vi "Obtain Request Events.vi"(8 "error in (no error)":errorcluster, 10 "Create New? (F)":bool) -> (0 "error out":errorcluster, 2 "Acquisition Request Events":T1)   [LabVIEW 2019, in "Acquisition.lvlib"]
doc: "This VI Obtains/Creates the Requests events that will be used for other modules to communicate with the module that owns this VI. These Requests events will be accessed only via Public API methods for this module.\n\n<b>NOTE</b>: The contents of this VI are automatically generated and modified by the <b>Tools > Delacor > DQMH</b> utilities. Consider using those utilities instead of making your own modifications to this VI.\n_____\nBased on Delacor QMH Project Template 4.0.0.47.\n_____\nBased on DQMH Project Template 6.1.0.94."
uses:
  Acquisition.lvlib
  Request Events--cluster.ctl
  Stop Argument--cluster.ctl
  Show Panel Argument--cluster.ctl
  Hide Panel Argument--cluster.ctl
  Get Module Execution Status Argument--cluster.ctl
  Show Diagram Argument--cluster.ctl
  Stop Acquiring Argument--cluster.ctl
  Wakeup Helper Loop Argument--cluster.ctl
  WiBCI16T_Data.ctl
  WiBCI16T_Status.ctl
  Reg_Map.ctl
  Acquisition Types.ctl
  Change Settings Argument--cluster.ctl
  Signal Type--enum.ctl
  Calibration Values--cluster.ctl
  Calibrate DAQ Argument--cluster.ctl
  Start Acquiring Argument--cluster.ctl
  Start Acquiring (Reply Payload)--cluster.ctl
  Command_TestData Argument--cluster.ctl
  Check WiFi AP Argument--cluster.ctl
  Command_NoiseData Argument--cluster.ctl
  Command_LiveData Argument--cluster.ctl
  Command_ImpedanceData Argument--cluster.ctl
  Command_GoToIdle Argument--cluster.ctl
  Soft Trigger Argument--cluster.ctl
  Start IMP Acquiring Argument--cluster.ctl
  Stop IMP acquiring Argument--cluster.ctl
  Start GND Loop acquiring Argument--cluster.ctl
  IMP data updated Argument--cluster.ctl
  IMP data updated (Reply Payload)--cluster.ctl
  Start CNV Acquiring Argument--cluster.ctl
  Start EOC Acquiring Argument--cluster.ctl
  Wake-up Helper Loop for Pkt Loss Calc Argument--cluster.ctl
  Stop Pkt Loss Calc Argument--cluster.ctl
  Update Packet ID Argument--cluster.ctl
  Calculate Packet Loss Argument--cluster.ctl
  Command_GndImpedanceData Argument--cluster.ctl
panel:
  # "NOTE: The contents of this VI are automatically generated and modified by the Tools > Delacor > DQMH utilities. Consider using those utilities instead of making your own modifications to this VI."
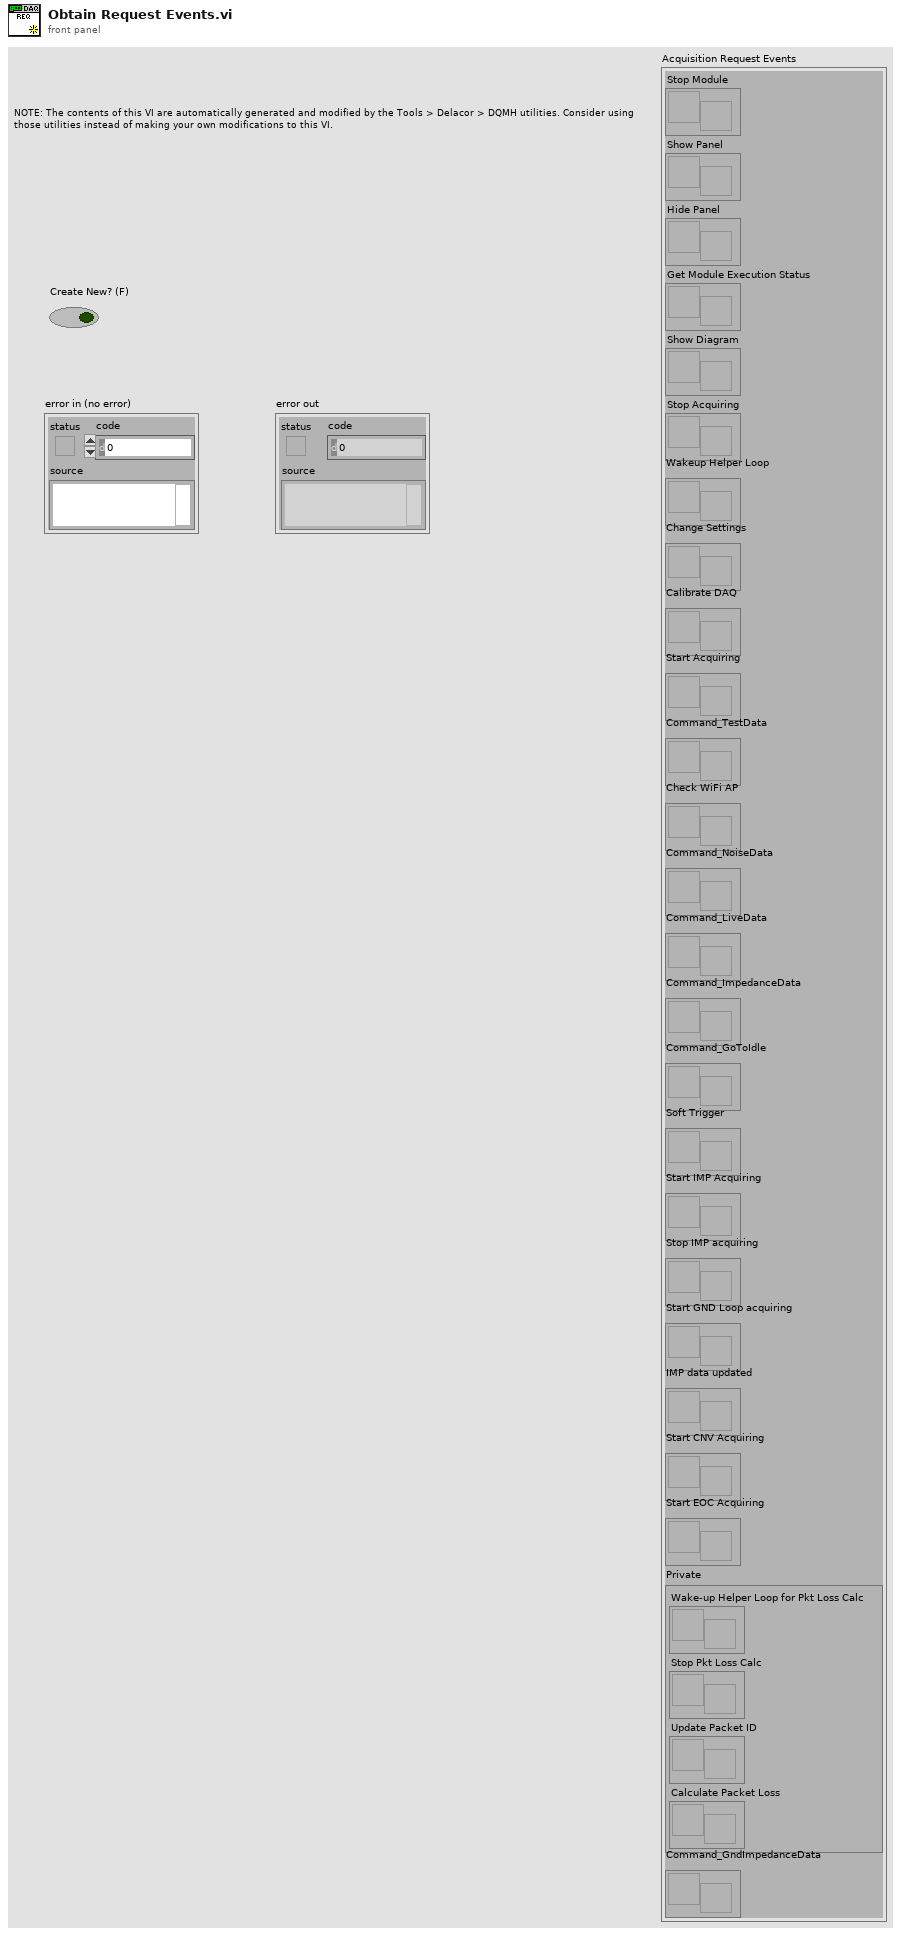
[diagram p1: front panel]
types:
  T1 = typedef "Acquisition.lvlib/Request Events--cluster.ctl" = cluster{"Stop Module":refnum<user-event>, "Show Panel":refnum<user-event>, "Hide Panel":refnum<user-event>, "Get Module Execution Status":refnum<user-event>, "Show Diagram":refnum<user-event>, "Stop Acquiring":refnum<user-event>, "Wakeup Helper Loop":refnum<user-event>, "Change Settings":refnum<user-event>, "Calibrate DAQ":refnum<user-event>, "Start Acquiring":refnum<user-event>, "Command_TestData":refnum<user-event>, "Check WiFi AP":refnum<user-event>, "Command_NoiseData":refnum<user-event>, "Command_LiveData":refnum<user-event>, "Command_ImpedanceData":refnum<user-event>, "Command_GoToIdle":refnum<user-event>, "Soft Trigger":refnum<user-event>, "Start IMP Acquiring":refnum<user-event>, "Stop IMP acquiring":refnum<user-event>, "Start GND Loop acquiring":refnum<user-event>, "IMP data updated":refnum<user-event>, "Start CNV Acquiring":refnum<user-event>, "Start EOC Acquiring":refnum<user-event>, "Private":cluster{"Wake-up Helper Loop for Pkt Loss Calc":refnum<user-event>, "Stop Pkt Loss Calc":refnum<user-event>, "Update Packet ID":refnum<user-event>, "Calculate Packet Loss":refnum<user-event>}, "Command_GndImpedanceData":refnum<user-event>}
  T2 = typedef "Acquisition.lvlib/Command_GndImpedanceData Argument--cluster.ctl" = cluster{"Boolean":bool}
  T3 = typedef "Acquisition.lvlib/Calculate Packet Loss Argument--cluster.ctl" = cluster{"Data Array":u32[]}
  T4 = typedef "Acquisition.lvlib/Update Packet ID Argument--cluster.ctl" = cluster{"Packet ID":u32}
  T5 = typedef "Acquisition.lvlib/Stop Pkt Loss Calc Argument--cluster.ctl" = cluster{"Boolean":bool}
  T6 = typedef "Acquisition.lvlib/Wake-up Helper Loop for Pkt Loss Calc Argument--cluster.ctl" = cluster{"Boolean":bool}
  T7 = typedef "Acquisition.lvlib/Start EOC Acquiring Argument--cluster.ctl" = cluster{"Boolean":bool}
  T8 = typedef "Acquisition.lvlib/Start CNV Acquiring Argument--cluster.ctl" = cluster{"Boolean":bool}
  T9 = typedef "Acquisition.lvlib/IMP data updated Argument--cluster.ctl" = cluster{"Wait Notifier":refnum<notifier>, "wait for reply":bool}
  T10 = typedef "Acquisition.lvlib/Start GND Loop acquiring Argument--cluster.ctl" = cluster{"Boolean":bool}
  T11 = typedef "Acquisition.lvlib/Stop IMP acquiring Argument--cluster.ctl" = cluster{"Boolean":bool}
  T12 = typedef "Acquisition.lvlib/Start IMP Acquiring Argument--cluster.ctl" = cluster{"Boolean":bool}
  T13 = typedef "Acquisition.lvlib/Soft Trigger Argument--cluster.ctl" = cluster{"Value":i8}
  T14 = typedef "Acquisition.lvlib/Command_GoToIdle Argument--cluster.ctl" = cluster{"Boolean":bool}
  T15 = typedef "Acquisition.lvlib/Command_ImpedanceData Argument--cluster.ctl" = cluster{"Boolean":bool}
  T16 = typedef "Acquisition.lvlib/Command_LiveData Argument--cluster.ctl" = cluster{"Boolean":bool}
  T17 = typedef "Acquisition.lvlib/Command_NoiseData Argument--cluster.ctl" = cluster{"Boolean":bool}
  T18 = typedef "Acquisition.lvlib/Check WiFi AP Argument--cluster.ctl" = cluster{"Connected ?":bool}
  T19 = typedef "Acquisition.lvlib/Command_TestData Argument--cluster.ctl" = cluster{"Boolean":bool}
  T20 = typedef "Acquisition.lvlib/Start Acquiring Argument--cluster.ctl" = cluster{"Wait Notifier":refnum<notifier>, "wait for reply":bool}
  T21 = typedef "Acquisition.lvlib/Calibrate DAQ Argument--cluster.ctl" = cluster{"None":bool}
  T22 = typedef "Acquisition.lvlib/Change Settings Argument--cluster.ctl" = cluster{"Signal Type":T23, "Calibration Array":T24[]}
  T23 = typedef "Acquisition.lvlib/Signal Type--enum.ctl" = enum16{"Sine Wave", "Square with Noise"}
  T24 = typedef "Acquisition.lvlib/Calibration Values--cluster.ctl" = cluster{"Slope":dbl, "Offset":dbl}
  T25 = typedef "Acquisition.lvlib/Wakeup Helper Loop Argument--cluster.ctl" = cluster{"connection UDP":refnum<k16>, "En MAP":u16, "WiBCI16T Data out":T26, "Acquisition Types":T29}
  T26 = typedef "Acquisition.lvlib/WiBCI16T_Data.ctl" = cluster{"EEG Ch 1":dbl, "EEG Ch 2":dbl, "EEG Ch 3":dbl, "EEG Ch 4":dbl, "EEG Ch 5":dbl, "EEG Ch 6":dbl, "EEG Ch 7":dbl, "EEG Ch 8":dbl, "EEG Ch 9":dbl, "EEG Ch 10":dbl, "EEG Ch 11":dbl, "EEG Ch 12":dbl, "EEG Ch 13":dbl, "EEG Ch 14":dbl, "EEG Ch 15":dbl, "EEG Ch 16":dbl, "X-Accel":i16, "Y-Accel":i16, "Z-Accel":i16, "X-Gyro":i16, "Y-Gyro":i16, "Z-Gyro":i16, "Timer":u32, "Packet ID":u32, "HW Trig1":u8, "SW Trig1":i8, "HW Trig2":u8, "SW Trig2":i8, "WiBCI Status":T27, "Reg Map":T28}
  T27 = typedef "Acquisition.lvlib/WiBCI16T_Status.ctl" = cluster{"Mode Byte":u8, "Ch Config":u8, "Ch Ref Map":u16, "Ch Enable Map":u16, "Temperature":sgl, "Battery":u8, "Version":string}
  T28 = typedef "Acquisition.lvlib/Reg_Map.ctl" = cluster{"ADS1":u8[], "ADS2":u8[]}
  T29 = typedef "Acquisition.lvlib/Acquisition Types.ctl" = cluster{"Acq Types":enum16{"Single Graph", "Eyes O/C", "CNV Demo", "Impedance", "Graph"}}
  T30 = typedef "Acquisition.lvlib/Stop Acquiring Argument--cluster.ctl" = cluster{"Boolean":bool}
  T31 = typedef "Acquisition.lvlib/Hide Panel Argument--cluster.ctl" = cluster{"Hide Panel?":bool}
  T32 = typedef "Acquisition.lvlib/Show Panel Argument--cluster.ctl" = cluster{"Show Panel?":bool}
  T33 = typedef "Acquisition.lvlib/Show Diagram Argument--cluster.ctl" = cluster{"Debug?":bool}
  T34 = typedef "Acquisition.lvlib/Get Module Execution Status Argument--cluster.ctl" = cluster{"Running?":bool}
  T35 = typedef "Acquisition.lvlib/Stop Argument--cluster.ctl" = cluster{"Origin":string, "Exit via Stop Module Req?":bool, "Wait for Module to stop?":bool}
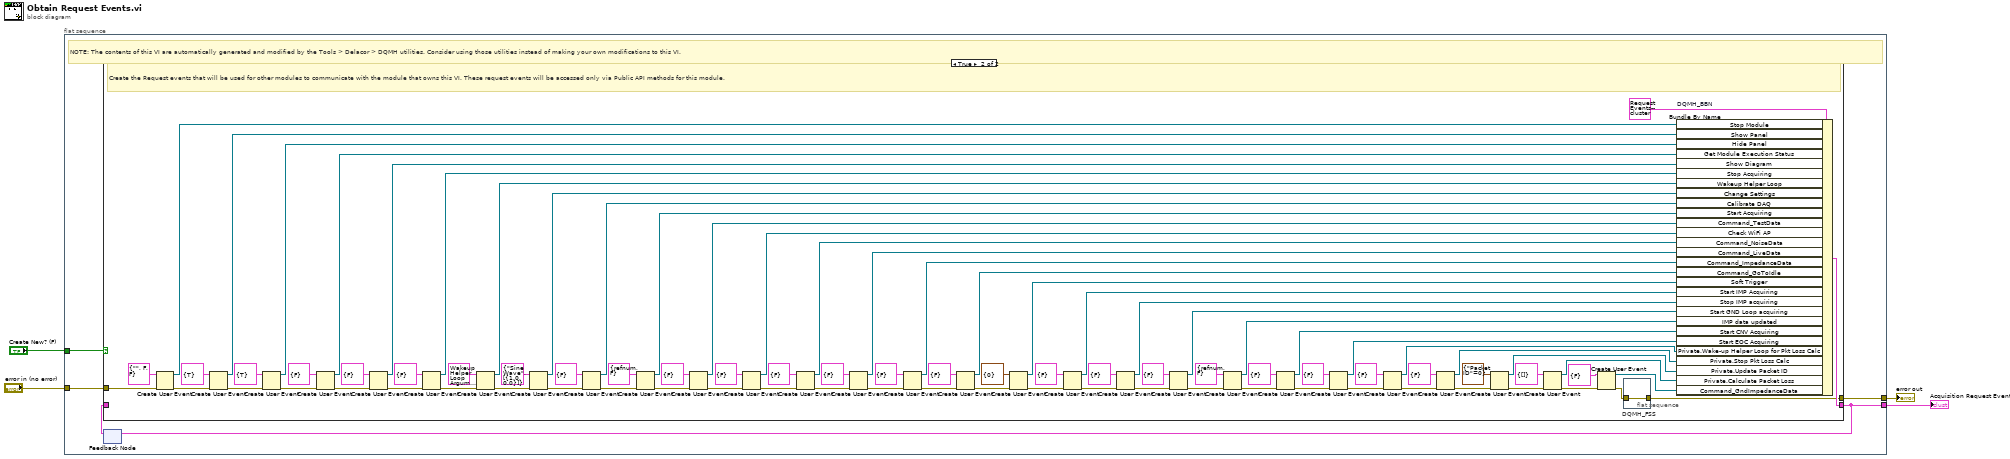
[diagram p0: block diagram]
diagram:
  n1 = flat-sequence {
    tunnel: [w9] -> w4
    tunnel: "error in (no error)" -> [w8]
    tunnel: [w6] -> w2
    tunnel: "Create New? (F)" -> [w5]
    frame #0 {
      # "NOTE: The contents of this VI are automatically generated and modified by the Tools > Delacor > DQMH utilities. Consider using those utilities instead of making your own modifications to this VI."
      n2 = feedback #1() -> (w7:T1)  [unwired: 1 in]
      n3 = case shown="True" w5 {
        tunnel: [w10 w89] -> w9
        tunnel: w8 -> [w10 w99]
        tunnel: [w11 w96] -> w6
        tunnel: w7 -> [w11 _]
        frame False {
          # "Obtain the Request events that were created in a previous call to this VI."
        }
        frame True {
          # "Create the Request events that will be used for other modules to communicate with the module that owns this VI. These request events will be accessed only via Public API methods for this module."
          n4 = Create User Event(user event datatype=T35 {"Origin"="", "Exit via Stop Module Req?"=FALSE, "Wait for Module to stop?"=FALSE} ("Stop Argument"), error in=w99) -> (user event=w97:refnum<user-event>, error out=w94:errorcluster)
          n5 = Create User Event(user event datatype=T32 {"Show Panel?"=TRUE} ("Show Panel Argument"), error in=w94) -> (user event=w93:refnum<user-event>, error out=w92:errorcluster)
          n6 = Create User Event(user event datatype=T31 {"Hide Panel?"=TRUE} ("Hide Panel Argument"), error in=w92) -> (user event=w91:refnum<user-event>, error out=w90:errorcluster)
          n7 = Create User Event(user event datatype=T34 {"Running?"=FALSE} ("Get Module Execution Status Argument"), error in=w90) -> (user event=w87:refnum<user-event>, error out=w88:errorcluster)
          n8 = Create User Event(user event datatype=T33 {"Debug?"=FALSE} ("Show Diagram Argument"), error in=w88) -> (user event=w84:refnum<user-event>, error out=w85:errorcluster)
          n9 = Create User Event(user event datatype=T30 {"Boolean"=FALSE} ("Stop Acquiring Argument"), error in=w85) -> (user event=w79:refnum<user-event>, error out=w80:errorcluster)
          n10 = Create User Event(user event datatype=T25 {"connection UDP"=refnum, "En MAP"=0, "WiBCI16T Data out"={"EEG Ch 1"=0.0, "EEG Ch 2"=0.0, "EEG Ch 3"=0.0, "EEG Ch 4"=0.0, "EEG Ch 5"=0.0, "EEG Ch 6"=0.0, "EEG Ch 7"=0.0, "EEG Ch 8"=0.0, "EEG Ch 9"=0.0, "EEG Ch 10"=0.0, "EEG Ch 11"=0.0, "EEG Ch 12"=0.0, "EEG Ch 13"=0.0, "EEG Ch 14"=0.0, "EEG Ch 15"=0.0, "EEG Ch 16"=0.0, "X-Accel"=0, "Y-Accel"=0, "Z-Accel"=0, "X-Gyro"=0, "Y-Gyro"=0, "Z-Gyro"=0, "Timer"=0, "Packet ID"=0, "HW Trig1"=0, "SW Trig1"=0, "HW Trig2"=0, "SW Trig2"=0, "WiBCI Status"={"Mode Byte"=0, "Ch Config"=0, "Ch Ref Map"=0, "Ch Enable Map"=0, "Temperature"=0.0, "Battery"=0, "Version"=""}, "Reg Map"={"ADS1"=[], "ADS2"=[]}}, "Acquisition Types"={"Acq Types"=enum."Single Graph"}} ("Wakeup Message Pump Argument"), error in=w80) -> (user event=w76:refnum<user-event>, error out=w77:errorcluster)
          n11 = Create User Event(user event datatype=T22 {"Signal Type"=enum."Sine Wave", "Calibration Array"=[{"Slope"=1.0, "Offset"=0.0}]} ("Change Settings Argument"), error in=w77) -> (user event=w73:refnum<user-event>, error out=w74:errorcluster)
          n12 = Create User Event(user event datatype=T21 {"None"=FALSE} ("Calibrate DAQ Argument"), error in=w74) -> (user event=w70:refnum<user-event>, error out=w71:errorcluster)
          n13 = Create User Event(user event datatype=T20 {"Wait Notifier"=refnum, "wait for reply"=FALSE} ("Start Acquisition Argument"), error in=w71) -> (user event=w67:refnum<user-event>, error out=w68:errorcluster)
          n14 = Create User Event(user event datatype=T19 {"Boolean"=FALSE} ("Command_TestData Argument"), error in=w68) -> (user event=w64:refnum<user-event>, error out=w65:errorcluster)
          n15 = Create User Event(user event datatype=T18 {"Connected ?"=FALSE} ("Check WiFi AP Argument"), error in=w65) -> (user event=w61:refnum<user-event>, error out=w62:errorcluster)
          n16 = Create User Event(user event datatype=T17 {"Boolean"=FALSE} ("Command_NoiseData Argument"), error in=w62) -> (user event=w58:refnum<user-event>, error out=w59:errorcluster)
          n17 = Create User Event(user event datatype=T16 {"Boolean"=FALSE} ("Command_LiveData Argument"), error in=w59) -> (user event=w55:refnum<user-event>, error out=w56:errorcluster)
          n18 = Create User Event(user event datatype=T15 {"Boolean"=FALSE} ("Command_ImpedanceData Argument"), error in=w56) -> (user event=w52:refnum<user-event>, error out=w53:errorcluster)
          n19 = Create User Event(user event datatype=T14 {"Boolean"=FALSE} ("Command_GoToIdle Argument"), error in=w53) -> (user event=w49:refnum<user-event>, error out=w50:errorcluster)
          n20 = Create User Event(user event datatype=T13 {"Value"=0} ("Soft Trigger Argument"), error in=w50) -> (user event=w46:refnum<user-event>, error out=w47:errorcluster)
          n21 = Create User Event(user event datatype=T12 {"Boolean"=FALSE} ("Start IMP Acquiring Argument"), error in=w47) -> (user event=w43:refnum<user-event>, error out=w44:errorcluster)
          n22 = Create User Event(user event datatype=T11 {"Boolean"=FALSE} ("Stop IMP acquiring Argument"), error in=w44) -> (user event=w40:refnum<user-event>, error out=w41:errorcluster)
          n23 = Create User Event(user event datatype=T10 {"Boolean"=FALSE} ("Start GND Loop acquiring Argument"), error in=w41) -> (user event=w37:refnum<user-event>, error out=w38:errorcluster)
          n24 = Create User Event(user event datatype=T9 {"Wait Notifier"=refnum, "wait for reply"=FALSE} ("IMP data updated Argument"), error in=w38) -> (user event=w34:refnum<user-event>, error out=w35:errorcluster)
          n25 = Create User Event(user event datatype=T8 {"Boolean"=FALSE} ("Start CNV Acquiring Argument"), error in=w35) -> (user event=w31:refnum<user-event>, error out=w32:errorcluster)
          n26 = Create User Event(user event datatype=T7 {"Boolean"=FALSE} ("Start EOC Acquiring Argument"), error in=w32) -> (user event=w28:refnum<user-event>, error out=w29:errorcluster)
          n27 = Create User Event(user event datatype=T6 {"Boolean"=FALSE} ("Wake-up Helper Loop for Pkt Loss Calc Argument"), error in=w29) -> (user event=w25:refnum<user-event>, error out=w26:errorcluster)
          n28 = Create User Event(user event datatype=T5 {"Boolean"=FALSE} ("Stop Pkt Loss Calc Argument"), error in=w26) -> (user event=w22:refnum<user-event>, error out=w23:errorcluster)
          n29 = Create User Event(user event datatype=T4 {"Packet ID"=0} ("Update Packet ID Argument"), error in=w23) -> (user event=w19:refnum<user-event>, error out=w20:errorcluster)
          n30 = Create User Event(user event datatype=T3 {"Data Array"=[]} ("Calculate Packet Loss Argument"), error in=w20) -> (user event=w16:refnum<user-event>, error out=w17:errorcluster)
          n31 = Create User Event(user event datatype=T2 {"Boolean"=FALSE} ("Command_GndImpedanceData Argument"), error in=w17) -> (user event=w13:refnum<user-event>, error out=w14:errorcluster)
          n32 = flat-sequence "DQMH_FSS" {
            tunnel: w14 -> [w100]
            tunnel: [w100] -> w89
            frame #0 {
            }
          }
          n33 = Bundle By Name "DQMH_BBN"(cluster=T1 {"Stop Module"=refnum, "Show Panel"=refnum, "Hide Panel"=refnum, "Get Module Execution Status"=refnum, "Show Diagram"=refnum, "Stop Acquiring"=refnum, "Wakeup Helper Loop"=refnum, "Change Settings"=refnum, "Calibrate DAQ"=refnum, "Start Acquiring"=refnum, "Command_TestData"=refnum, "Check WiFi AP"=refnum, "Command_NoiseData"=refnum, "Command_LiveData"=refnum, "Command_ImpedanceData"=refnum, "Command_GoToIdle"=refnum, "Soft Trigger"=refnum, "Start IMP Acquiring"=refnum, "Stop IMP acquiring"=refnum, "Start GND Loop acquiring"=refnum, "IMP data updated"=refnum, "Start CNV Acquiring"=refnum, "Start EOC Acquiring"=refnum, "Private"={"Wake-up Helper Loop for Pkt Loss Calc"=refnum, "Stop Pkt Loss Calc"=refnum, "Update Packet ID"=refnum, "Calculate Packet Loss"=refnum}, "Command_GndImpedanceData"=refnum} ("output cluster"), "Stop Module"=w97, "Show Panel"=w93, "Hide Panel"=w91, "Get Module Execution Status"=w87, "Show Diagram"=w84, "Stop Acquiring"=w79, "Wakeup Helper Loop"=w76, "Change Settings"=w73, "Calibrate DAQ"=w70, "Start Acquiring"=w67, "Command_TestData"=w64, "Check WiFi AP"=w61, "Command_NoiseData"=w58, "Command_LiveData"=w55, "Command_ImpedanceData"=w52, "Command_GoToIdle"=w49, "Soft Trigger"=w46, "Start IMP Acquiring"=w43, "Stop IMP acquiring"=w40, "Start GND Loop acquiring"=w37, "IMP data updated"=w34, "Start CNV Acquiring"=w31, "Start EOC Acquiring"=w28, "Private.Wake-up Helper Loop for Pkt Loss Calc"=w25, "Private.Stop Pkt Loss Calc"=w22, "Private.Update Packet ID"=w19, "Private.Calculate Packet Loss"=w16, "Command_GndImpedanceData"=w13) -> (w96:T1)
        }
      }
      n34 = feedback-in #1(w6) -> ()
    }
  }
  "Acquisition Request Events" <- w2
  "error out" <- w4
